vi "RichToFlatni_bus_monitor_api_StopProcessRequest.vi"(5 "OutputClusterType":T1, 11 "InputCluster":T3) -> (3 "OutputCluster":T1)   [LabVIEW 2025, in "bus_monitor_server.lvlib"]
uses:
  bus_monitor_server.lvlib
  ni_bus_monitor_api_StopProcessRequest.ctl
  ni_bus_monitor_api_Session.ctl
  ni_bus_monitor_api_StopProcessRequest_Flat.ctl
  ni_bus_monitor_api_Session_Flat.ctl
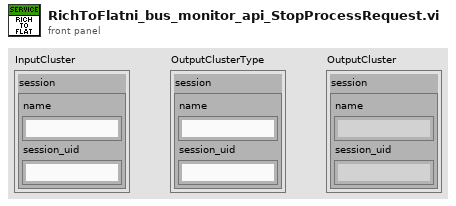
[diagram p1: front panel]
types:
  T1 = typedef "bus_monitor_server.lvlib/ni_bus_monitor_api_StopProcessRequest_Flat.ctl" = cluster{"session":T2}
  T2 = typedef "bus_monitor_server.lvlib/ni_bus_monitor_api_Session_Flat.ctl" = cluster{"name":string, "session_uid":string}
  T3 = typedef "bus_monitor_server.lvlib/ni_bus_monitor_api_StopProcessRequest.ctl" = cluster{"session":T4}
  T4 = typedef "bus_monitor_server.lvlib/ni_bus_monitor_api_Session.ctl" = cluster{"name":string, "session_uid":string}
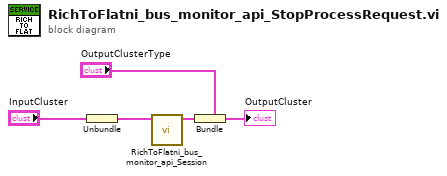
[diagram p0: block diagram]
diagram:
  n1 = Unbundle "Unbundle"("InputCluster") -> ("session"=w2:T4)
  n2 = call "RichToFlatni_bus_monitor_api_Session.vi"("InputCluster"=w2) -> ("OutputCluster"=w1:T2)  [unwired: 10 in]
  n3 = Bundle "Bundle"(cluster="OutputClusterType", "session"=w1) -> (→"OutputCluster":T1)
